vi "getConfig.vi"() -> ()   [LabVIEW 2023, in "CCD.lvclass"]
uses:
  CCD.lvclass
  CCD.lvclass/CCD.ctl
  20f7d3bd-08ac-4524-9bed-df36c1da25a0.vi
  a21955fc-e3a0-4e36-8495-41f1bfac7860.vi
  GenericDevice/GenericDevice.lvclass
panel:
  out "CCD out":refnum<class "CCD.lvclass">
  in  "CCD in":refnum<class "CCD.lvclass">
  out "error out":errorcluster
  in  "error in (no error)":errorcluster
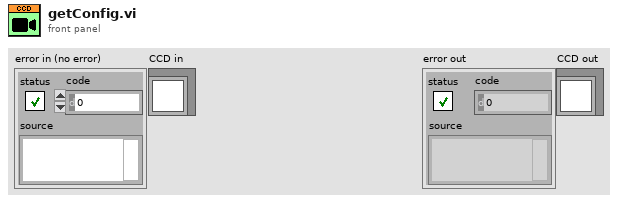
[diagram p1: front panel]
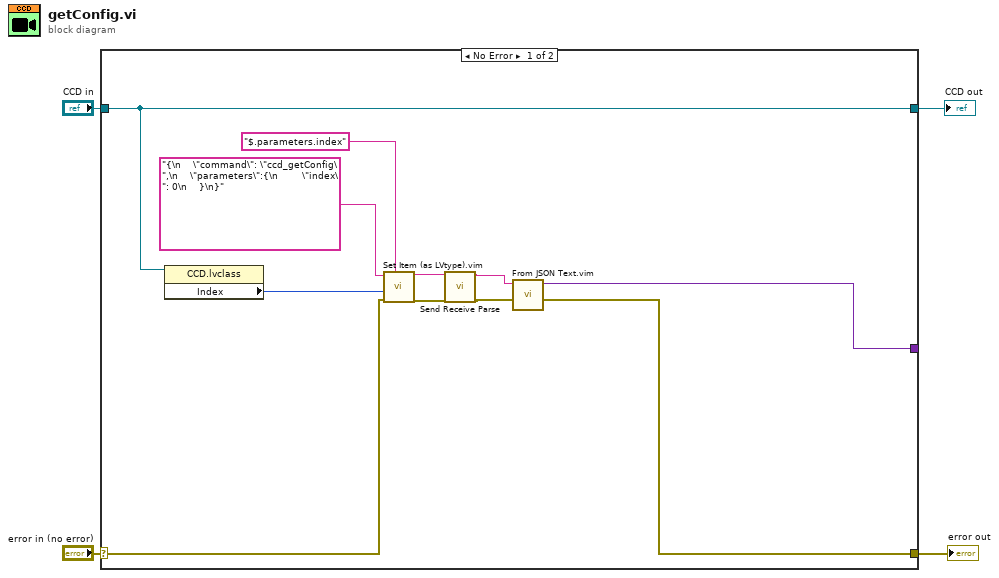
[diagram p0: block diagram]
diagram:
  n1 = case shown="No Error" "error in (no error)" {
    selector: "error in (no error)" -> [w11 w17]
    tunnel: [w9 w17] -> w3
    tunnel: [w13 w16] -> w1
    tunnel: "CCD in" -> [w13 w16]
    tunnel: [w10 _] -> _
    frame No Error {
      n2 = property class="CCD.lvclass"(reference=w13) -> ("Index"=w12:i32)  [unwired: 1 in, 2 out]
      n3 = call "Set Item (as LVtype).vim"("$Path or Item Name"="$.parameters.index", "error in (no error)"=w11, "Anything"=w12, "JSON"="{\n    \"command\": \"ccd_getConfig\",\n    \"parameters\":{\n        \"index\": 0\n    }\n}") -> ("error out"=w6:errorcluster, "<JSON>"=w8:string)  [unwired: 4 in, 1 out]
      n4 = call "Send Receive Parse.vi"("<JSON>"=w8, "error in"=w6) -> ("results-JSON string"=w7:string, "error out"=w5:errorcluster)  [unwired: 9 in, 7 out]
      n5 = call "From JSON Text.vim"("error in (no error)"=w5, "JSON"=w7) -> ("error out"=w9:errorcluster, "Data out"=w10:variant)  [unwired: 8 in]
    }
    frame Error {
    }
  }
  "error out" <- w3
  "CCD out" <- w1
